vi "set_maximum_output_value.vi"(8 "error in (no error)":errorcluster, 10 "maximum output value":dbl, 11 "GenericWriteSignals.lvclass in":refnum<class "SignalWriterMH110203USBStepperMotor.lvclass">) -> (0 "error out":errorcluster, 3 "GenericWriteSignals.lvclass out":refnum<class "SignalWriterMH110203USBStepperMotor.lvclass">)   [LabVIEW 2010, in "SignalWriterMH110203USBStepperMotor.lvclass"]
uses:
  SignalWriterMH110203USBStepperMotor.lvclass
  SignalWriterMH110203USBStepperMotor.lvclass/SignalWriterMH110203USBStepperMotor.ctl
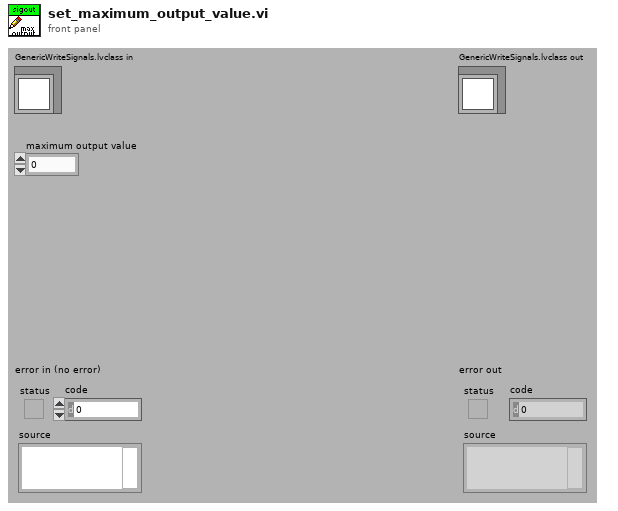
[diagram p1: front panel]
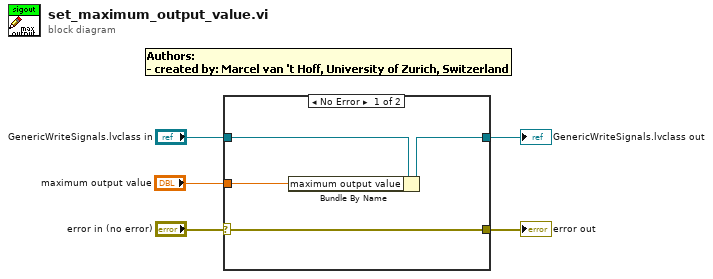
[diagram p0: block diagram]
diagram:
  n1 = case shown="No Error" "error in (no error)" {
    selector: "error in (no error)" -> [w9 w10]
    tunnel: [w9 w10] -> w2
    tunnel: [w7 w11] -> w1
    tunnel: "GenericWriteSignals.lvclass in" -> [w8 w11]
    tunnel: "maximum output value" -> [w6 _]
    frame No Error {
      n2 = Bundle By Name(cluster=w8, "maximum output value"=w6) -> (w7:refnum<class "SignalWriterMH110203USBStepperMotor.lvclass">)
    }
    frame Error {
    }
  }
  "error out" <- w2
  "GenericWriteSignals.lvclass out" <- w1
